vi "Render_AD_Results.vi"(4 "Background Color":u32(colorbox)=16448250, 5 "Rel._Margin":sgl=0.2, 8 "error in":errorcluster, 11 "Anomaly Detection Rresults":T1={"Image"="remote image 000001443E0F18B8", "Ground Truth"="remote image 000001443E0F3018", "Predicted Heat Map"="remote image 000001443E0F25C8", "Predicted Mask"="remote image 000001443E0F1808", "Segmentation"="remote image 000001443E0F2E08"}) -> (0 "error out":errorcluster, 3 "Anomaly Detection Results":T2(plugin-control))   [LabVIEW 2024]
uses:
  Controls/Anomaly_Detection_Results_Imgs.ctl
  <vilib>/vision/NI_Vision_Development_Module.lvlib
panel:
  out "Font Size 2":i16
  out "Font Size":i16
  in  "Desired Font (Application)":T3(ring)
  in  "[User-specified Font].Font Name":string="system font"
  in  "Horizontal Alignment":i16(ring)=1 items=["Left", "Center", "Right"]
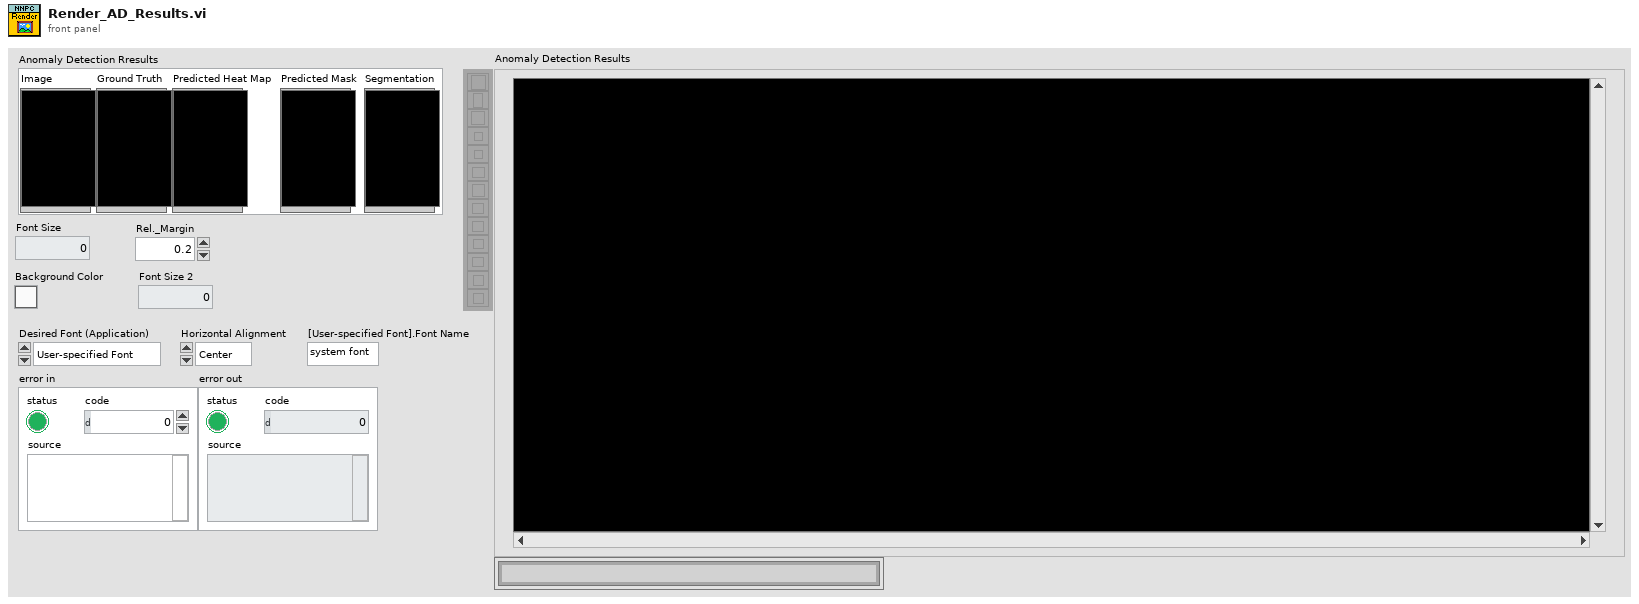
[diagram p1: front panel]
types:
  T1 = typedef "Anomaly_Detection_Results_Imgs.ctl" = cluster{"Image":T2, "Ground Truth":T2, "Predicted Heat Map":T2, "Predicted Mask":T2, "Segmentation":T2}
  T2 = typedef "IMAQ Image.ctl" = refnum<image>
  T3 = enum16{"User-specified Font", "Application Font", "System Font", "Dialog Font"}
  T4 = cluster{"Desired Font (Application)":enum16{"User-specified Font", "Application Font", "System Font", "Dialog Font"}, "[User-specified Font]":cluster{"Font Name":string, "Size":i16, "Strikeout?":bool, "Italic?":bool, "Underline?":bool, "Outline?":bool, "Shadow?":bool, "Bold?":bool, "Rotation Angle":dbl}, "Horizontal Alignment":i16, "Vertical Alignment":i16}
  T5 = typedef "Image Type" = u32
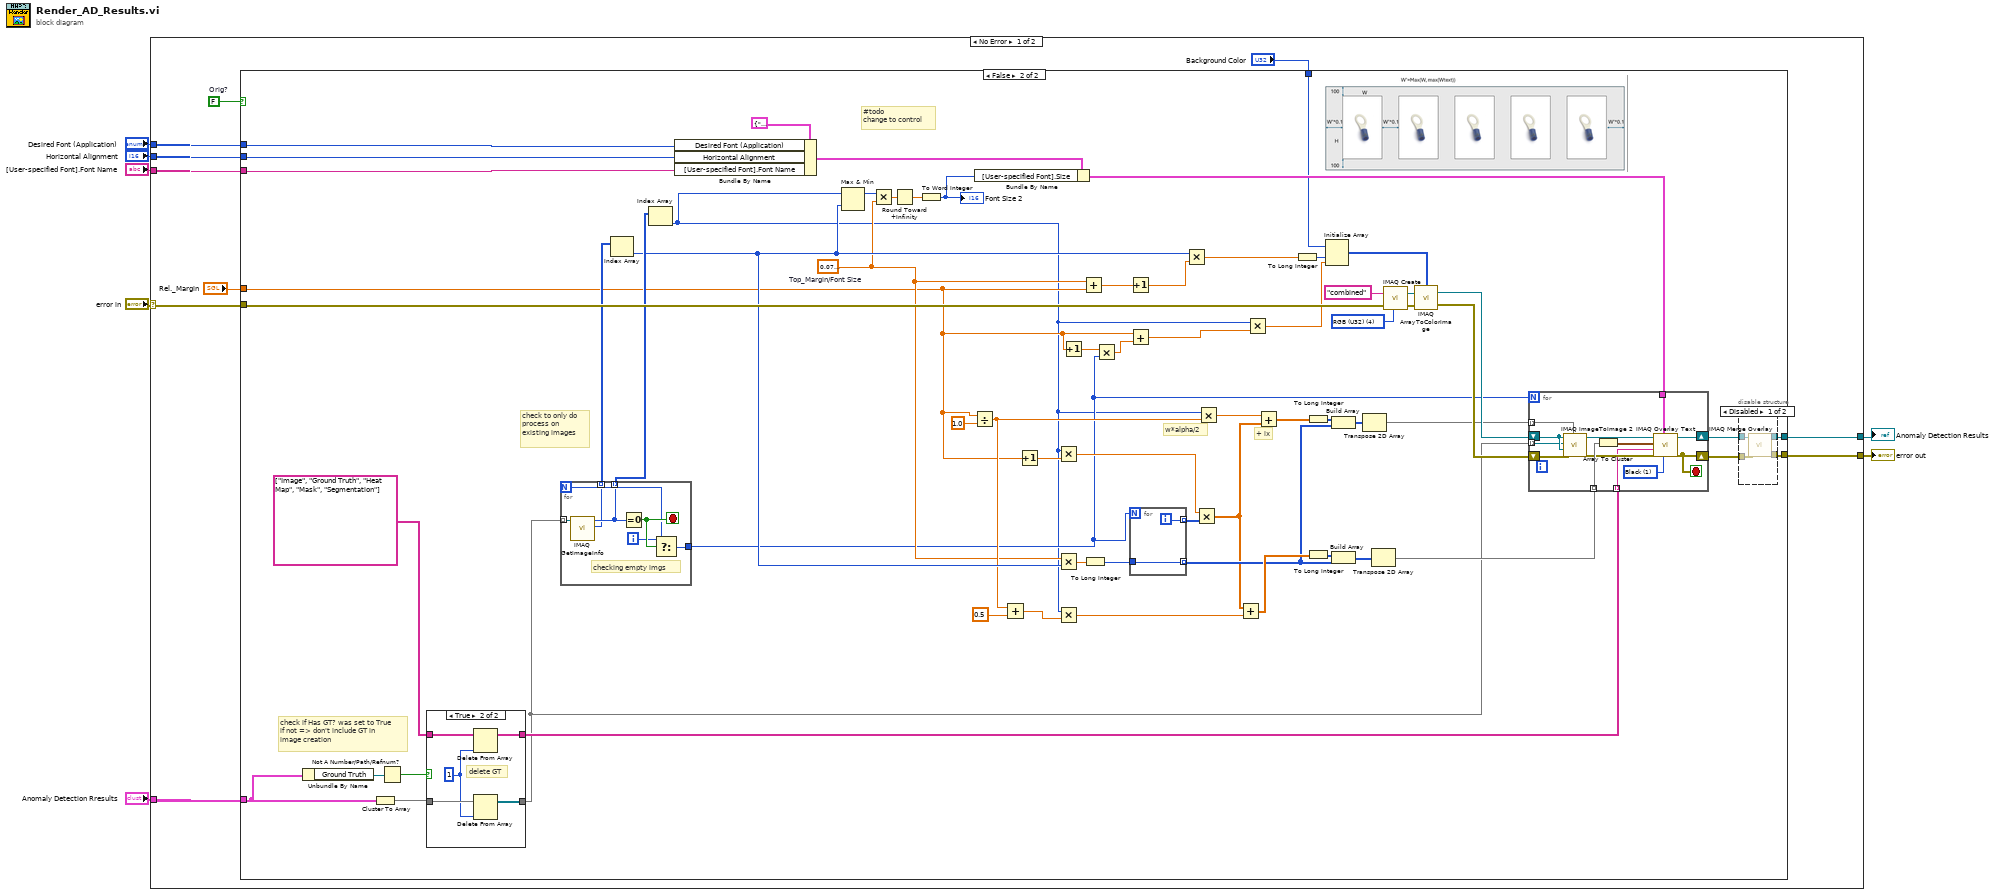
[diagram p0: block diagram]
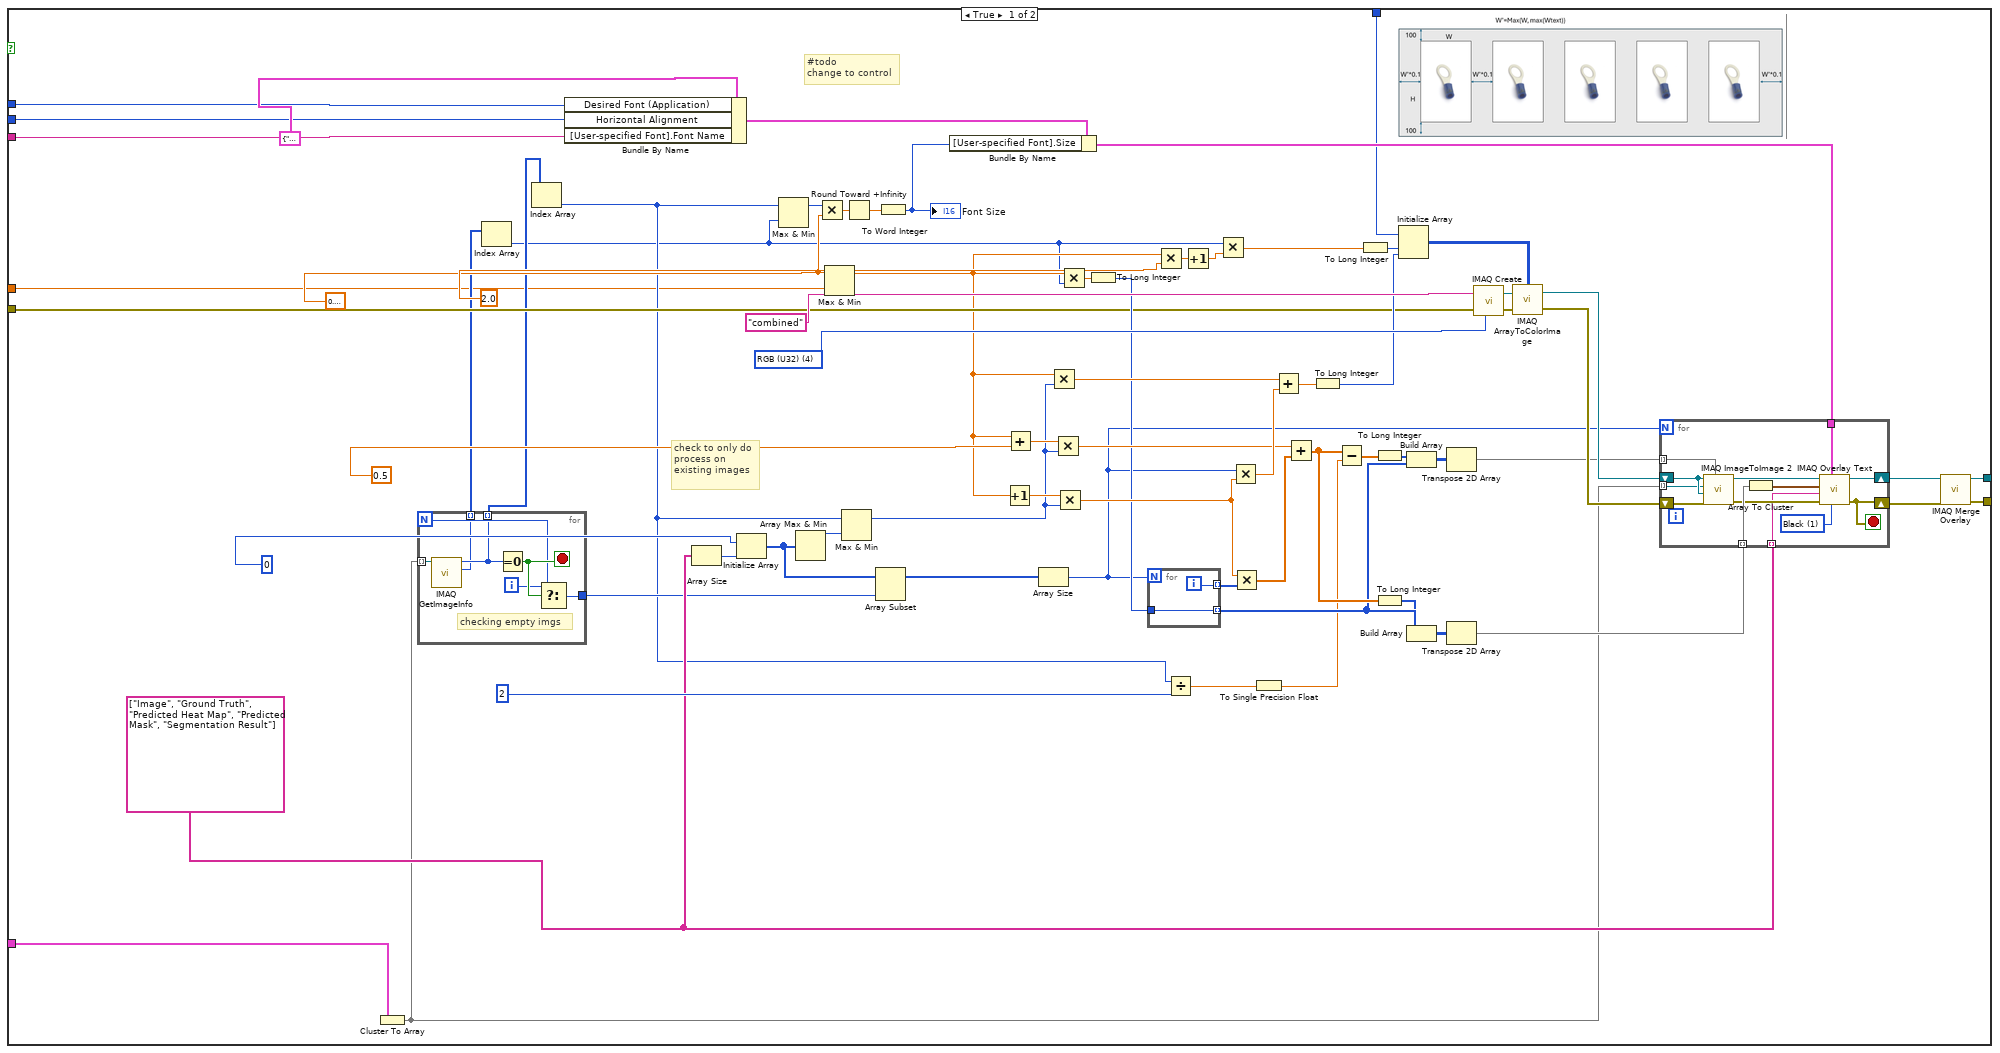
[diagram p2: hidden frame]
diagram:
  n1 = case shown="No Error" "error in" {
    selector: "error in" -> [w13 w212]
    tunnel: "Horizontal Alignment" -> [w17 _]
    tunnel: "[User-specified Font].Font Name" -> [w16 _]
    tunnel: "Desired Font (Application)" -> [w15 _]
    tunnel: [w11 w212] -> w1
    tunnel: [w12 _] -> w2
    tunnel: "Anomaly Detection Rresults" -> [w14 _]
    frame No Error {
      w10 = FALSE  # Orig?
      n2 = case shown="False" w10 {
        tunnel: w17 -> [w79 w168]
        tunnel: w16 -> [w74 w167]
        tunnel: w15 -> [w73 w166]
        tunnel: w14 -> [w43 w122]
        tunnel: w13 -> [w42 w150]
        tunnel: [w27 w144] -> w12
        tunnel: [w25 w142] -> w11
        tunnel: "Rel._Margin" -> [w19 w115]
        tunnel: "Background Color" -> [w18 w137]
        frame True {
          w33 = sgl 0.1 ("y")
          w46 = string[] ["Image", "Ground Truth", "Predicted Heat Map", "Predicted Mask", "Segmentation Result"] ("String")
          w88 = T5 4 items=["Grayscale (U8)", "Grayscale (I16)", "Grayscale (SGL)", "Complex (CSG)", "RGB (U32)", "HSL (U32)", "RGB (U64)", "Grayscale (U16)"] ("Image Type")
          # "#todo\nchange to control"
          # "check to only do process on existing images"
          n3 = Cluster To Array(cluster=w43) -> (array=w41:T2[])
          n4 = for {
            N -> [w93]
            tunnel: w41 -> [w97] mode=indexing
            tunnel: [w96] -> w28
            tunnel: [w92] -> w23 mode=indexing
            tunnel: [w91] -> w22 mode=indexing
            i -> [w94]
            stop <- w95 stop-if-true
            # "checking empty imgs"
            n5 = call "IMAQ GetImageInfo"("Image"=w97) -> ("Y Resolution"=w91:i32, "X Resolution"=w92:i32)  [unwired: 3 in, 6 out]
            n6 = Equal To 0?(x=w92) -> (x = 0?=w95:bool)
            n7 = Select(t=w94, s=w95, f=w93) -> (s? t:f=w96:i32)
          }
          n8 = Index Array(array=w22) -> (element=w20:i32)  [unwired: 1 in]
          n9 = Index Array(array=w23) -> (element=w21:i32)  [unwired: 1 in]
          n10 = Bundle By Name(cluster=T4 {"Desired Font (Application)"=enum."Application Font", "[User-specified Font]"={"Font Name"="", "Size"=12, "Strikeout?"=FALSE, "Italic?"=FALSE, "Underline?"=FALSE, "Outline?"=FALSE, "Shadow?"=FALSE, "Bold?"=FALSE, "Rotation Angle"=0.0}, "Horizontal Alignment"=0, "Vertical Alignment"=0} ("Font, Size & Style"), "Desired Font (Application)"=w73, "Horizontal Alignment"=w79, "[User-specified Font].Font Name"=w74) -> (w38:T4)
          n11 = Array Size(array=w46) -> (size(s)=w29:i32)
          n12 = Initialize Array(0 ("String width"), w29) -> (w36:i32[])
          n13 = Max & Min(x=w21, y=w20) -> (max(x,y)=w45:i32)  [unwired: 1 out]
          n14 = Array Max & Min(array=w36) -> (max value=w83:i32)  [unwired: 3 out]
          n15 = Multiply(x=w45, y=w33) -> (x*y=w44:sgl)
          n16 = Max & Min(x=w33, y=w19) -> (max(x,y)=w32:sgl)  [unwired: 1 out]
          n17 = Max & Min(x=w21, y=w83) -> (max(x,y)=w56:i32)  [unwired: 1 out]
          n18 = Round Toward +Infinity(x=w44) -> (ceil(x): smallest int >= x=w35:sgl)
          n19 = Array Subset(array=w36, length=w28) -> (w40:i32[])  [unwired: 1 in]
          n20 = To Word Integer(number=w35) -> (16bit integer=w31:i16)
          "Font Size" <- w31
          n21 = Bundle By Name(cluster=w38, "[User-specified Font].Size"=w31) -> (w37:T4)
          n22 = Increment(x=w32) -> (x+1=w61:sgl)
          n23 = Add(x=w32, y=sgl 0.5) -> (x+y=w57:sgl)
          n24 = Array Size(array=w40) -> (size(s)=w39:i32)
          n25 = Multiply(x=w32, y=w56) -> (x*y=w60:sgl)
          n26 = Multiply(x=w57, y=w56) -> (x*y=w55:sgl)
          n27 = Multiply(x=w61, y=w56) -> (x*y=w59:sgl)
          n28 = Multiply(x=w32, y=w20) -> (x*y=w34:sgl)
          n29 = To Long Integer(number=w34) -> (32bit integer=w47:i32)
          n30 = for {
            N: w39 -> [_]
            tunnel: [w90] -> w69 mode=indexing
            tunnel: [w89] -> w66 mode=indexing
            tunnel: w47 -> [w89]
            i -> [w90]
          }
          n31 = Multiply(x=w32, y=sgl 2.0) -> (x*y=w77:sgl)
          n32 = Divide(x=w21, y=2) -> (x/y=w65:dbl)
          n33 = Increment(x=w77) -> (x+1=w49:sgl)
          n34 = Multiply(x=w20, y=w49) -> (x*y=w75:sgl)
          n35 = Multiply(x=w39, y=w59) -> (x*y=w63:sgl)
          n36 = Multiply(x=w59, y=w69) -> (x*y=w68:sgl[])
          n37 = To Single Precision Float(number=w65) -> (single precision float=w50:sgl)
          n38 = Add(x=w60, y=w63) -> (x+y=w70:sgl)
          n39 = Add(x=w55, y=w68) -> (x+y=w67:sgl[])
          n40 = To Long Integer(number=w70) -> (32bit integer=w62:i32)
          n41 = Subtract(x=w67, y=w50) -> (x-y=w64:sgl[])
          n42 = To Long Integer(number=w75) -> (32bit integer=w48:i32)
          n43 = To Long Integer(number=w64) -> (32bit integer=w51:i32[])
          n44 = To Long Integer(number=w67) -> (32bit integer=w52:i32[])
          n45 = Initialize Array(w18, w48, w62) -> (w86:u32[][])
          n46 = Build Array(w51, w66) -> (w82:i32[][])
          n47 = Build Array(w52, w66) -> (w81:i32[][])
          n48 = Transpose 2D Array(2D array=w82) -> (transposed array=w54:i32[][])
          n49 = Transpose 2D Array(2D array=w81) -> (transposed array=w53:i32[][])
          n50 = call "IMAQ Create"("Image Name"="combined", "Image Type"=w88, "error in (no error)"=w42) -> ("New Image"=w85:T2, "error out"=w72:errorcluster)  [unwired: 2 in]
          n51 = call "IMAQ ArrayToColorImage"("Image Pixels (U32)"=w86, "Image"=w85, "error in (no error)"=w72) -> ("Image Out"=w84:T2, "error out"=w71:errorcluster)  [unwired: 2 in]
          n52 = for {
            N: w39 -> [_]
            tunnel: w41 -> [w108] mode=indexing
            shift-right: [w105] -> w24
            shift-left: w84 -> [w109]
            tunnel: w46 -> [w101] mode=indexing
            tunnel: w54 -> [w110] mode=indexing
            tunnel: w53 -> [w104] mode=indexing
            tunnel: w37 -> [w103]
            shift-right: [w100] -> w26
            shift-left: w71 -> [w107]
            stop <- w100 stop-if-true
            w99 = 1 items=["White", "Black", "Inverted", "Black on White", "White on Black"] ("Color")
            n53 = call "IMAQ ImageToImage 2"("Offset Left/Top"=w110, "error in (no error)"=w107, "Image Dst"=w109, "Image Src (Small)"=w108, "Image Src (Large)"=w109) -> ("error out"=w102:errorcluster, "Image Dst Out"=w106:T2)  [unwired: 5 in]
            n54 = Array To Cluster(array=w104) -> (cluster=w98:cluster{"[0]":i32, "[1]":i32})
            n55 = call "IMAQ Overlay Text"("Text Color (black)"=w99, "Font, Size & Style"=w103, "error in (no error)"=w102, "String"=w101, "Origin"=w98, "Image"=w106) -> ("error out"=w100:errorcluster, "Image Out"=w105:T2)  [unwired: 4 in]
          }
          n56 = call "IMAQ Merge Overlay"("error in (no error)"=w26, "Image Src"=w24) -> ("error out"=w25:errorcluster, "Image Dst Out"=w27:T2)  [unwired: 8 in]
        }
        frame False {
          w118 = sgl 0.08  # Top_Margin/Font Size
          w176 = T5 4 items=["Grayscale (U8)", "Grayscale (I16)", "Grayscale (SGL)", "Complex (CSG)", "RGB (U32)", "HSL (U32)", "RGB (U64)", "Grayscale (U16)"] ("Image Type")
          # "check if Has GT? was set to True\nif not => don't include GT in \nimage creation"
          # "+ ix"
          # "w*alpha/2"
          # "#todo\nchange to control"
          # "check to only do process on existing images"
          n57 = Unbundle By Name(w122) -> ("Ground Truth"=w126:T2)
          n58 = Cluster To Array(cluster=w122) -> (array=w121:T2[])
          n59 = Not A Number/Path/Refnum?(number/path/refnum=w126) -> (NaN/Path/Refnum?=w125:bool)
          n60 = case shown="True" w125 {
            tunnel: w121 -> [w205 w211]
            tunnel: [w205 w208] -> w120
            tunnel: string[] ["Image", "Ground Truth", "Heat Map", "Mask", "Segmentation"] ("String") -> [w206 w210]
            tunnel: [w206 w209] -> w123
            frame False {
            }
            frame True {
              w207 = 1 ("index")
              # "delete GT"
              n61 = Delete From Array(array=w210, index=w207) -> (array with subset deleted=w209:string[])  [unwired: 1 in, 1 out]
              n62 = Delete From Array(array=w211, index=w207) -> (array with subset deleted=w208:T2[])  [unwired: 1 in, 1 out]
            }
          }
          n63 = for {
            N -> [w187]
            tunnel: w120 -> [w191] mode=indexing
            tunnel: [w190] -> w113
            tunnel: [w186] -> w140 mode=indexing
            tunnel: [w185] -> w139 mode=indexing
            i -> [w188]
            stop <- w189 stop-if-true
            # "checking empty imgs"
            n64 = call "IMAQ GetImageInfo"("Image"=w191) -> ("Y Resolution"=w185:i32, "X Resolution"=w186:i32)  [unwired: 3 in, 6 out]
            n65 = Equal To 0?(x=w186) -> (x = 0?=w189:bool)
            n66 = Select(t=w188, s=w189, f=w187) -> (s? t:f=w190:i32)
          }
          n67 = Index Array(array=w139) -> (element=w138:i32)  [unwired: 1 in]
          n68 = Index Array(array=w140) -> (element=w111:i32)  [unwired: 1 in]
          n69 = Bundle By Name(cluster=T4 {"Desired Font (Application)"=enum."Application Font", "[User-specified Font]"={"Font Name"="", "Size"=12, "Strikeout?"=FALSE, "Italic?"=FALSE, "Underline?"=FALSE, "Outline?"=FALSE, "Shadow?"=FALSE, "Bold?"=FALSE, "Rotation Angle"=0.0}, "Horizontal Alignment"=0, "Vertical Alignment"=0} ("Font, Size & Style"), "Desired Font (Application)"=w166, "Horizontal Alignment"=w168, "[User-specified Font].Font Name"=w167) -> (w149:T4)
          n70 = Max & Min(x=w111, y=w138) -> (max(x,y)=w152:i32)  [unwired: 1 out]
          n71 = Multiply(x=w152, y=w118) -> (x*y=w151:sgl)
          n72 = Round Toward +Infinity(x=w151) -> (ceil(x): smallest int >= x=w147:sgl)
          n73 = To Word Integer(number=w147) -> (16bit integer=w145:i16)
          "Font Size 2" <- w145
          n74 = Divide(x=w115, y=sgl 1.0) -> (x/y=w135:sgl)
          n75 = Bundle By Name(cluster=w149, "[User-specified Font].Size"=w145) -> (w148:T4)
          n76 = Add(x=w135, y=sgl 0.5) -> (x+y=w158:sgl)
          n77 = Increment(x=w115) -> (x+1=w160:sgl)
          n78 = Multiply(x=w111, y=w160) -> (x*y=w130:sgl)
          n79 = Multiply(x=w118, y=w138) -> (x*y=w146:sgl)
          n80 = Multiply(x=w111, y=w158) -> (x*y=w157:sgl)
          n81 = Increment(x=w115) -> (x+1=w116:sgl)
          n82 = Add(x=w118, y=w115) -> (x+y=w119:sgl)
          n83 = To Long Integer(number=w146) -> (32bit integer=w153:i32)
          n84 = Multiply(x=w116, y=w113) -> (x*y=w114:sgl)
          n85 = Increment(x=w119) -> (x+1=w117:sgl)
          n86 = Add(x=w115, y=w114) -> (x+y=w112:sgl)
          n87 = for {
            N: w113 -> [_]
            tunnel: [w184] -> w163 mode=indexing
            tunnel: [w183] -> w161 mode=indexing
            tunnel: w153 -> [w183]
            i -> [w184]
          }
          n88 = Multiply(x=w138, y=w117) -> (x*y=w128:sgl)
          n89 = Multiply(x=w130, y=w163) -> (x*y=w134:sgl[])
          n90 = Multiply(x=w111, y=w135) -> (x*y=w131:sgl)
          n91 = Add(x=w134, y=w157) -> (x+y=w162:sgl[])
          n92 = Multiply(x=w111, y=w112) -> (x*y=w129:sgl)
          n93 = Add(x=w131, y=w134) -> (x+y=w127:sgl[])
          n94 = To Long Integer(number=w128) -> (32bit integer=w154:i32)
          n95 = To Long Integer(number=w127) -> (32bit integer=w155:i32[])
          n96 = To Long Integer(number=w162) -> (32bit integer=w156:i32[])
          n97 = Initialize Array(w137, w154, w129) -> (w174:u32[][])
          n98 = Build Array(w155, w161) -> (w171:i32[][])
          n99 = Build Array(w156, w161) -> (w170:i32[][])
          n100 = Transpose 2D Array(2D array=w171) -> (transposed array=w132:i32[][])
          n101 = Transpose 2D Array(2D array=w170) -> (transposed array=w133:i32[][])
          n102 = call "IMAQ Create"("Image Name"="combined", "Image Type"=w176, "error in (no error)"=w150) -> ("New Image"=w173:T2, "error out"=w165:errorcluster)  [unwired: 2 in]
          n103 = call "IMAQ ArrayToColorImage"("Image Pixels (U32)"=w174, "Image"=w173, "error in (no error)"=w165) -> ("Image Out"=w172:T2, "error out"=w164:errorcluster)  [unwired: 2 in]
          n104 = for {
            N: w113 -> [_]
            tunnel: w120 -> [w203] mode=indexing
            shift-right: [w200] -> w141
            shift-left: w172 -> [w204]
            tunnel: w123 -> [w196] mode=indexing
            tunnel: w133 -> [w199] mode=indexing
            tunnel: w148 -> [w198]
            shift-right: [w195] -> w143
            shift-left: w164 -> [w202]
            tunnel: w132 -> [w192] mode=indexing
            stop <- w195 stop-if-true
            w194 = 1 items=["White", "Black", "Inverted", "Black on White", "White on Black"] ("Color")
            n105 = call "IMAQ ImageToImage 2"("Offset Left/Top"=w192, "error in (no error)"=w202, "Image Dst"=w204, "Image Src (Small)"=w203, "Image Src (Large)"=w204) -> ("error out"=w197:errorcluster, "Image Dst Out"=w201:T2)  [unwired: 5 in]
            n106 = Array To Cluster(array=w199) -> (cluster=w193:cluster{"[0]":i32, "[1]":i32})
            n107 = call "IMAQ Overlay Text"("Text Color (black)"=w194, "Font, Size & Style"=w198, "error in (no error)"=w197, "String"=w196, "Origin"=w193, "Image"=w201) -> ("error out"=w195:errorcluster, "Image Out"=w200:T2)  [unwired: 4 in]
          }
          n108 = disable-structure shown="Disabled" {
            disable-tunnel: [w180 w182] -> w144
            disable-tunnel: w143 -> [w179 w181]
            disable-tunnel: [w178 w181] -> w142
            disable-tunnel: w141 -> [w177 w182]
            frame Disabled {
              n109 = call "IMAQ Merge Overlay"("error in (no error)"=w179, "Image Src"=w177) -> ("error out"=w178:errorcluster, "Image Dst Out"=w180:T2)  [unwired: 8 in]
            }
            frame Enabled {
            }
          }
        }
      }
    }
    frame Error {
    }
  }
  "Anomaly Detection Results" <- w2
  "error out" <- w1
